vi "Keithley 6517A Display Config.vi"(3 "Display Enabled":bool=TRUE, 4 "Text To Display on Line 2":string, 5 "Display Text on Line 2":bool, 6 "error in":T1, 7 "Text To Display on Line 1":string, 8 "Display Text on Line 1":bool, 9 "GPIB address":string="27") -> (0 "error out":T1)   [LabVIEW 2013]
doc: "This VI is used to configure the display. The VI allows you to put messages up on the display, turn the display off, or display normal readings.\n\nGPIB Address: default = 27\n\nDisplay Text on Line 1:\nFALSE = Off\nTRUE = On\n\nText To Display on Line 1: Up to 20 characters\n\nDisplay Text on Line 2:\nFALSE = Off\nTRUE = On\n\nText To Display on Line 2: Up to 20 characters\n\nDisplayed Resolution: 4 to 7\n\nDisplay Enabled:\nFALSE = Off\nTRUE = On"
panel:
  # "ON\nOFF"
  # "ON\nOFF"
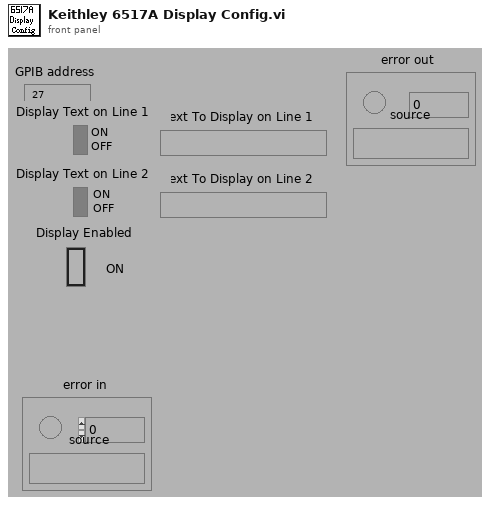
[diagram p1: front panel]
types:
  T1 = cluster{"error":bool, "code":i32, "source":string}
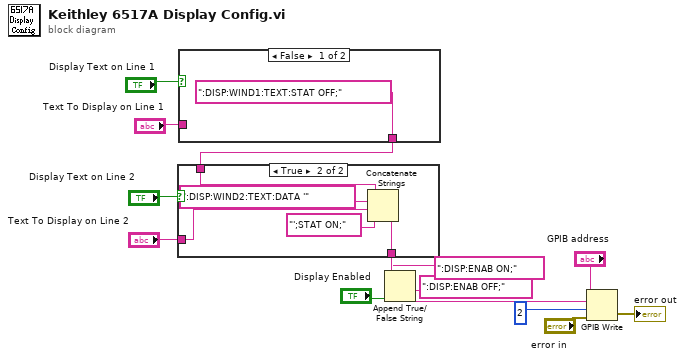
[diagram p0: block diagram]
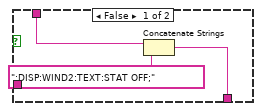
[diagram p2: hidden frame]
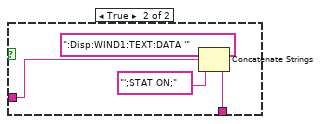
[diagram p3: hidden frame]
diagram:
  n1 = case shown="False" "Display Text on Line 1" {
    tunnel: "Text To Display on Line 1" -> [_ w18]
    tunnel: [":DISP:WIND1:TEXT:STAT OFF;" w16] -> w12
    frame False {
    }
    frame True {
      n2 = Concatenate Strings(":Disp:WIND1:TEXT:DATA '", w18, "';STAT ON;") -> (w16:string)
    }
  }
  n3 = case shown="True" "Display Text on Line 2" {
    tunnel: w12 -> [w21 w27]
    tunnel: "Text To Display on Line 2" -> [_ w25]
    tunnel: [w20 w23] -> w9
    frame False {
      n4 = Concatenate Strings(w21, ":DISP:WIND2:TEXT:STAT OFF;") -> (w20:string)
    }
    frame True {
      n5 = Concatenate Strings(w27, ":DISP:WIND2:TEXT:DATA '", w25, "';STAT ON;") -> (w23:string)
    }
  }
  n6 = Append True/False String(1:"Display Enabled", 2:":DISP:ENAB OFF;", 3:":DISP:ENAB ON;", 4:w9) -> (0:w4:string)
  n7 = GPIB Write(0:"GPIB address", 1:w4, 2:2, 3:"error in") -> (6:→"error out":errorcluster)  [unwired: 1 in, 1 out]
